vi "ADCP_Raw_To_Processed_Packet.vi"(8 "error in (no error)":errorcluster, 10 "Raw Packet":u8[](array[numeric]), 11 "ADCP in":refnum<class "ADCP.lvclass">) -> (0 "error out":errorcluster, 2 "Processed Packet":u8[](array[numeric]), 3 "ADCP out":refnum<class "ADCP.lvclass">)   [LabVIEW 2017, in "ADCP.lvclass"]
uses:
  ADCP.lvclass
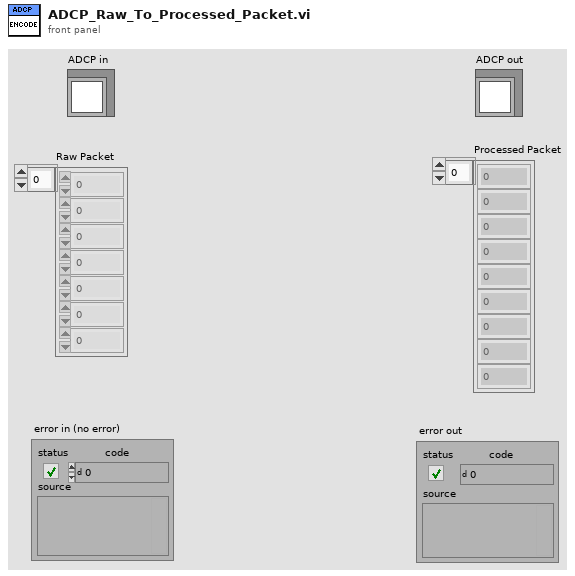
[diagram p1: front panel]
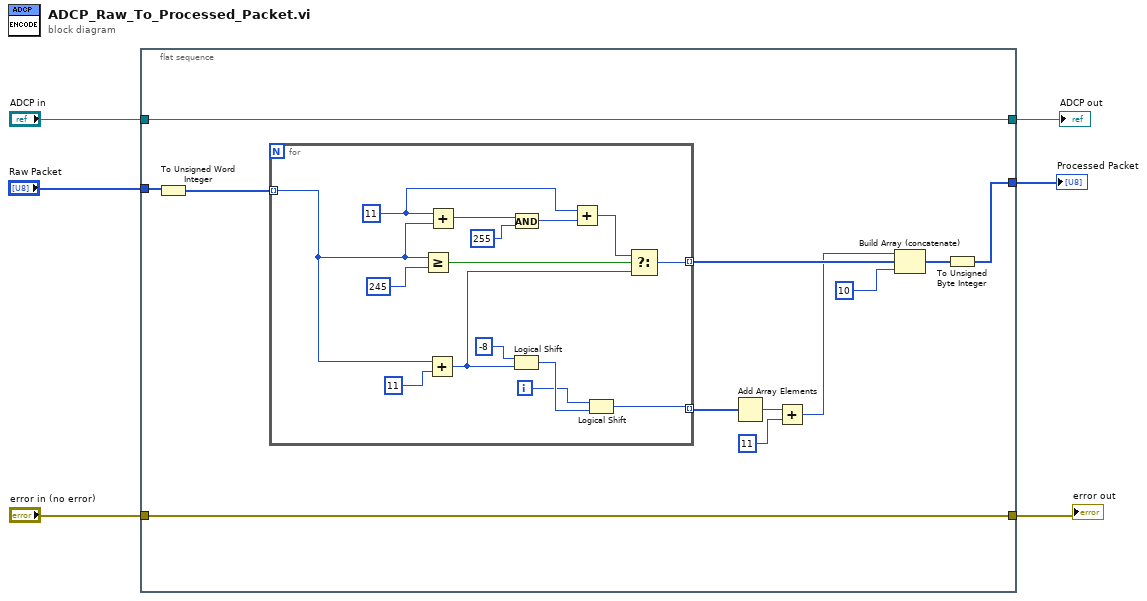
[diagram p0: block diagram]
diagram:
  n1 = flat-sequence {
    tunnel: "ADCP in" -> [w18]
    tunnel: [w18] -> w5
    tunnel: "Raw Packet" -> [w9]
    tunnel: "error in (no error)" -> [w8]
    tunnel: [w8] -> w2
    tunnel: [w7] -> w1
    frame #0 {
      n2 = To Unsigned Word Integer(number=w9) -> (unsigned 16bit integer=w17:u16[])
      n3 = for {
        tunnel: w17 -> [w25] mode=indexing
        tunnel: [w26] -> w15 mode=indexing
        tunnel: [w20] -> w16 mode=indexing
        i -> [w21]
        w28 = u16 11 ("x")
        n4 = Greater Or Equal?(x=w25, y=u16 245) -> (x >= y?=w32:bool)
        n5 = Add(x=w25, y=u16 11) -> (x+y=w19:u16)
        n6 = Add(x=w28, y=w25) -> (x+y=w31:u16)
        n7 = Logical Shift(y=i16 -8, x=w19) -> (x << y=w22:u16)
        n8 = And(x=w31, y=u16 255) -> (x .and. y?=w29:u16)
        n9 = Add(x=w28, y=w29) -> (x+y=w27:u16)
        n10 = Logical Shift(y=w21, x=w22) -> (x << y=w20:u16)
        n11 = Select(t=w27, s=w32, f=w19) -> (s? t:f=w26:u16)
      }
      n12 = Add Array Elements(numeric array=w16) -> (sum=w12:u16)
      n13 = Add(x=w12, y=u16 11) -> (x+y=w11:u16)
      n14 = Build Array (concatenate)(w11, w15, u16 10) -> (w13:u16[])
      n15 = To Unsigned Byte Integer(number=w13) -> (unsigned 8bit integer=w7:u8[])
    }
  }
  "error out" <- w2
  "Processed Packet" <- w1
  "ADCP out" <- w5
